vi "Modified Thompson Tau Test.vi"(9 "Multiplier":dbl=1.0 min=0.1 max=1000.0 step=0.01, 10 "Array in":dbl[](array[numeric])) -> (0 "% Outliers":dbl format="%#.2g%%", 1 "Outliers":dbl[](array[numeric]), 2 "Initia Array out":dbl[](array[numeric]), 3 "Array out without Outliers":dbl[](array[numeric]), 4 "Threshold":dbl)   [LabVIEW 2016]
doc: "This VI takes in a 1D array and calculate if there are any outliers based on the \"Modified Thompson Tau Test\"."
uses:
  <vilib>/gmath/statdist.llb/Student t Inverse CDF.vi
  <userlib>/_OpenG.lib/array/array.llb/Search 1D Array (DBL)__ogtk.vi
  <userlib>/_OpenG.lib/array/array.llb/Delete Elements from 1D Array (DBL)__ogtk.vi
  <vilib>/gmath/NI_Gmath.lvlib
panel:
  out "Considered Criteria":dbl[](array[numeric])
  out "Mean":dbl
  out "Current Criteria":dbl
  out "Inv CDF":dbl
  out "x*y":dbl
  out "Tau":dbl
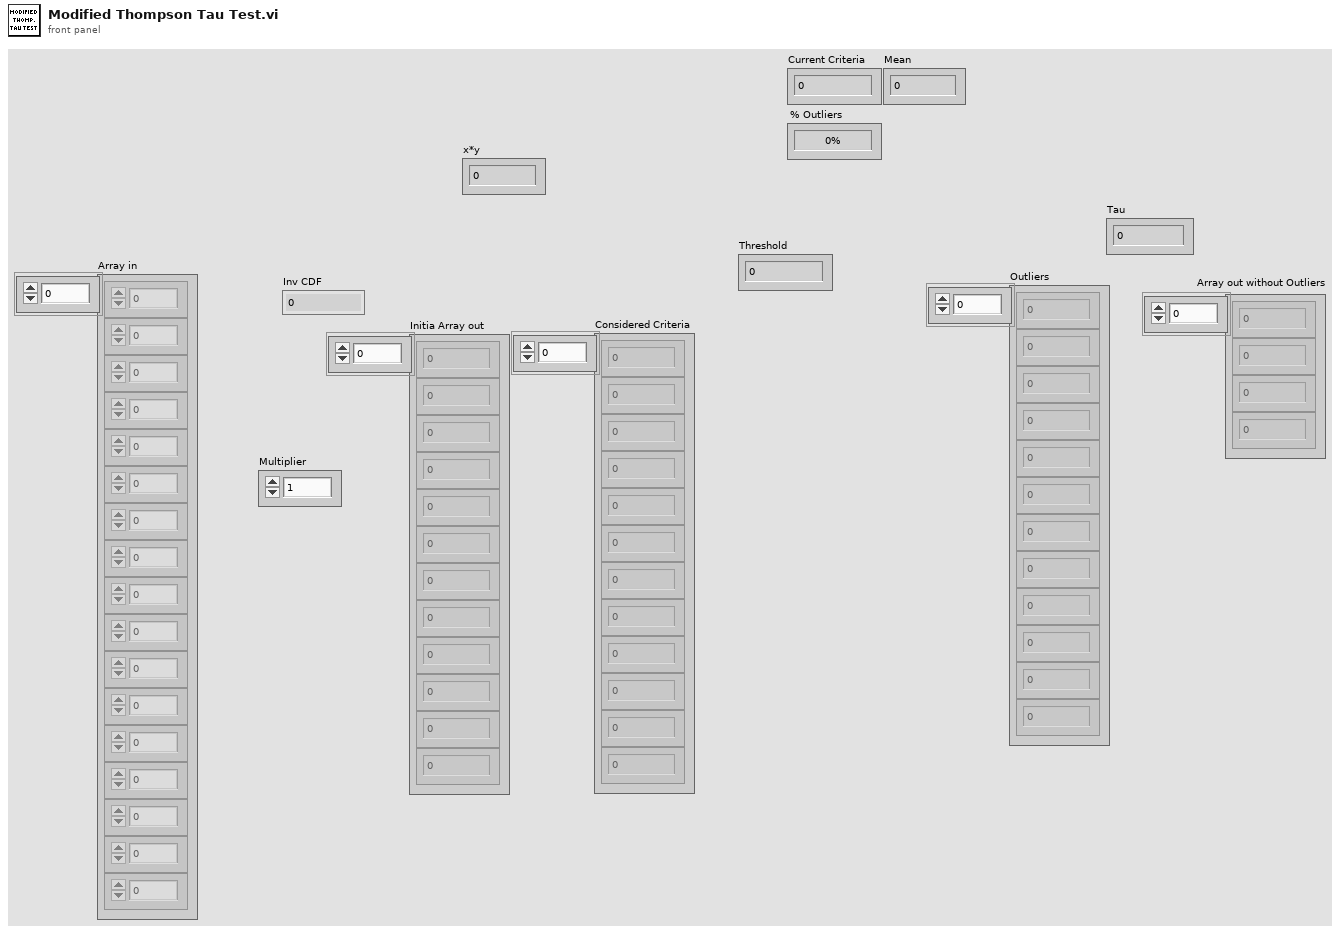
[diagram p1: front panel]
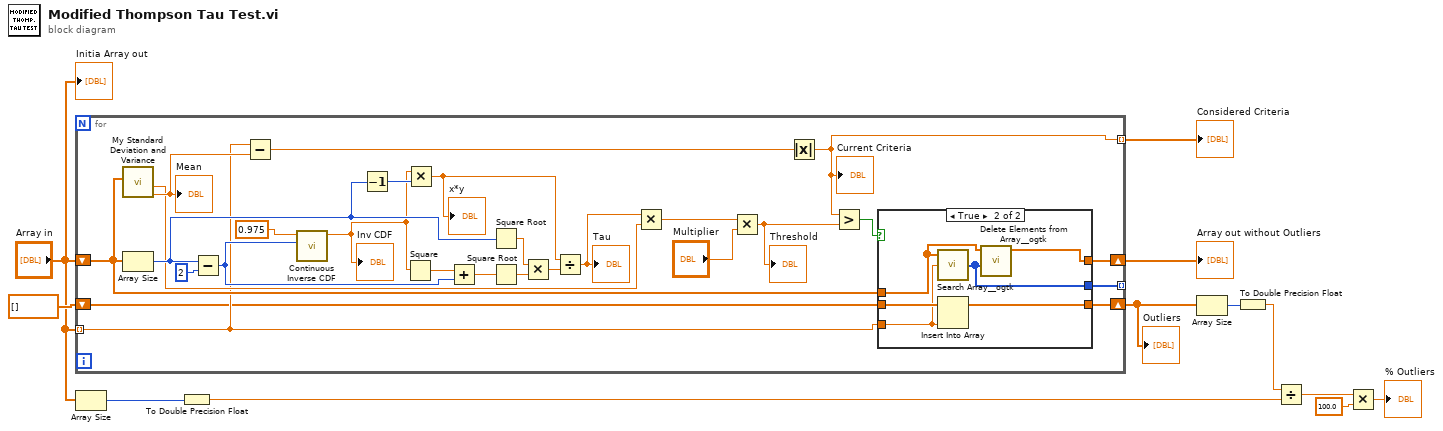
[diagram p0: block diagram]
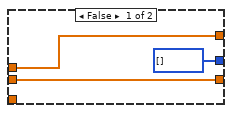
[diagram p2: hidden frame]
diagram:
  n1 = for {
    shift-right: [w21] -> w12
    shift-left: "Array in" -> [w22]
    tunnel: "Array in" -> [w20] mode=indexing
    tunnel: [w19] -> _ mode=indexing
    shift-right: [w17] -> w9
    shift-left: dbl[] [] ("sample set") -> [w18]
    tunnel: [w15] -> w10 mode=indexing
    n2 = call "My Standard Deviation and Variance.vi"("Array - Numeric"=w22) -> ("Mean"=w27:dbl, "Standard Deviation"=w24:dbl)  [unwired: 7 in, 2 out]
    "Mean" <- w27
    n3 = Array Size(array=w22) -> (size(s)=w36:i32)
    n4 = Subtract(x=w36, y=2) -> (x-y=w29:i32)
    n5 = Subtract(x=w20, y=w27) -> (x-y=w26:dbl)
    n6 = call-poly <vilib>:"Continuous Inverse CDF.vi"("k degrees of freedom"=w29, "cdf(x)"=0.975 ("x")) -> ("x"=w28:dbl)  [unwired: 8 in, 1 out]
    "Inv CDF" <- w28
    n7 = Decrement(x=w36) -> (x-1=w38:i32)
    n8 = Square(x=w28) -> (x^2=w34:dbl)
    n9 = Multiply(x=w28, y=w38) -> (x*y=w37:dbl)
    "x*y" <- w37
    n10 = Add(x=w34, y=w29) -> (x+y=w33:dbl)
    n11 = Square Root(x=w36) -> (sqrt(x)=w35:dbl)
    n12 = Square Root(x=w33) -> (sqrt(x)=w32:dbl)
    n13 = Multiply(x=w35, y=w32) -> (x*y=w31:dbl)
    n14 = Divide(x=w37, y=w31) -> (x/y=w25:dbl)
    "Tau" <- w25
    n15 = Multiply(x=w25, y=w24) -> (x*y=w14:dbl)
    n16 = Multiply(x=w14, y="Multiplier") -> (x*y=w13:dbl)
    "Threshold" <- w13
    n17 = Absolute Value(x=w26) -> (abs(x)=w15:dbl)
    "Current Criteria" <- w15
    n18 = Greater?(x=w15, y=w13) -> (0:w23:bool)
    n19 = case shown="True" w23 {
      tunnel: w22 -> [w42 w48]
      tunnel: [w42 w46] -> w21
      tunnel: w20 -> [_ w43]
      tunnel: [i32[] [] ("Indices of Elements") w47] -> w19
      tunnel: w18 -> [w40 w45]
      tunnel: [w40 w44] -> w17
      frame False {
      }
      frame True {
        n20 = call-poly <userlib>:"Search Array__ogtk.vi"("Array"=w48, "Element Data"=w43) -> ("Indices of Elements"=w47:i32[])  [unwired: 7 in]
        n21 = Insert Into Array(array=w45, new element=w43) -> (w44:dbl[])  [unwired: 1 in]
        n22 = call-poly <userlib>:"Delete Elements from Array__ogtk.vi"("indices"=w47, "array"=w48) -> ("array w/ subset deleted"=w46:dbl[])  [unwired: 8 in, 1 out]
      }
    }
  }
  "Array out without Outliers" <- w12
  "Outliers" <- w9
  "Considered Criteria" <- w10
  n23 = Array Size(array="Array in") -> (size(s)=w5:i32)
  n24 = To Double Precision Float(number=w5) -> (double precision float=w4:dbl)
  n25 = Array Size(array=w9) -> (size(s)=w7:i32)
  n26 = To Double Precision Float(number=w7) -> (double precision float=w6:dbl)
  n27 = Divide(x=w6, y=w4) -> (x/y=w3:dbl)
  n28 = Multiply(x=w3, y=100.0) -> (x*y=→"% Outliers":dbl)
  "Initia Array out" <- "Array in"
